vi "polling.vi"() -> ()   [LabVIEW 2026]
panel:
  out "Numeric":i32
  in  "stop":bool
  out "current time":timestamp
  in  "OK Button":bool
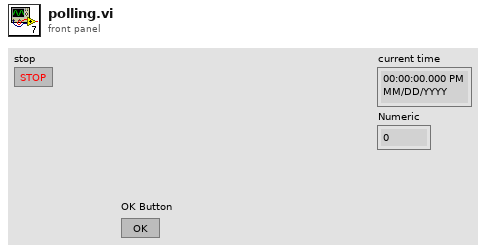
[diagram p1: front panel]
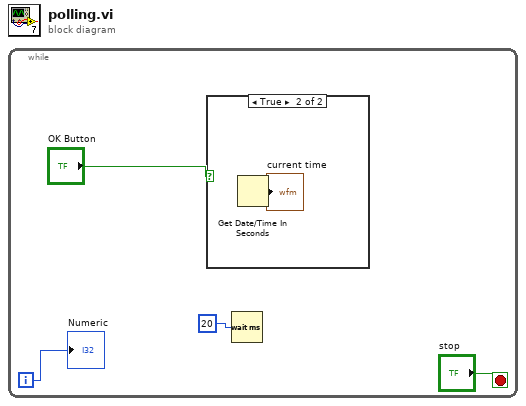
[diagram p0: block diagram]
diagram:
  n1 = while {
    i -> [w2]
    stop <- "stop" stop-if-true
    n2 = case shown="True" "OK Button" {
      frame False {
      }
      frame True {
        n3 = Get Date/Time In Seconds() -> (seconds since 1Jan1904=→"current time":timestamp)
      }
    }
    n4 = Wait (ms)(milliseconds to wait=u32 20) -> ()  [unwired: 1 out]
    "Numeric" <- w2
  }
